vi "Stop Core.vi"(10 "final error code":i32, 11 "Camera Controller in":refnum<class "Camera Controller.lvclass">) -> (3 "Camera Controller out":refnum<class "Camera Controller.lvclass">)   [LabVIEW 2019, in "Camera Controller.lvlib" / "Camera Controller.lvclass"]
doc: "(<B>Filename</B>: Actor Framework.lvlib:Actor.lvclass:Stop Core.vi)\n\nDefines what the actor does before it stops. Use the <B>final error code</B> input to determine whether the actor shut down in response to an error.\n\nBy default, this method does nothing. A descendant class may override it to define behavior, such as shutting down any processes the actor initiated in its override of the Actor Core method."
uses:
  Camera Controller.lvclass
  <vilib>/ActorFramework/Actor/Actor.lvclass
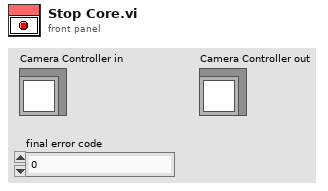
[diagram p1: front panel]
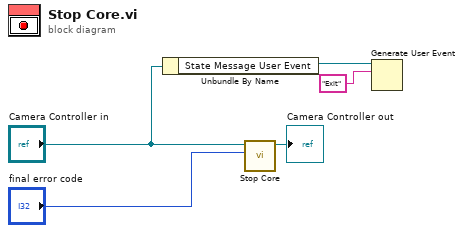
[diagram p0: block diagram]
diagram:
  n1 = Unbundle By Name("Camera Controller in") -> ("State Message User Event"=w2:refnum<user-event>)
  n2 = call-parent "Stop Core.vi"("final error code"="final error code", "Actor in"="Camera Controller in") -> ("Actor out"=→"Camera Controller out":refnum<class "Camera Controller.lvclass">)  [unwired: 9 in]
  n3 = Generate User Event(user event=w2, event data cluster="Exit" ("event data")) -> ()  [unwired: 2 in, 2 out]
